vi "Simulate CNT90.vi"(8 "error in (no error)":errorcluster, 10 "frec in":dbl=0.75 format="%#_13g", 11 "VISA resource name":refnum<visa-resource-name>) -> (0 "error out":errorcluster, 2 "Simulated Measurement":dbl, 3 "VISA resource name out":refnum<visa-resource-name>)   [LabVIEW 2019, in "CNT90.lvlib"]
uses:
  CNT90.lvlib
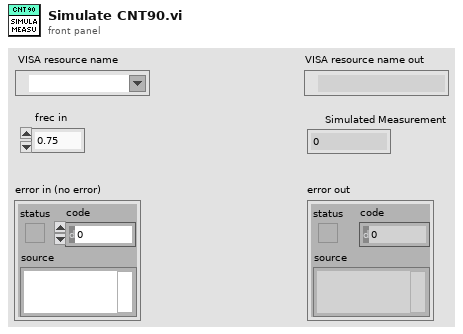
[diagram p1: front panel]
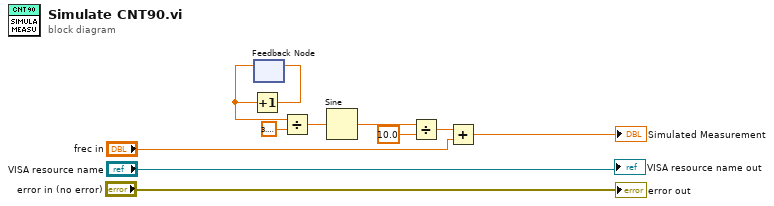
[diagram p0: block diagram]
diagram:
  n1 = feedback #1() -> (w7:dbl)  [unwired: 1 in]
  n2 = Increment(x=w7) -> (x+1=w11:dbl)
  n3 = feedback-in #1(w11) -> ()
  n4 = Divide(x=w7, y=3.141592653589793) -> (x/y=w10:dbl)
  n5 = Sine(x=w10) -> (sin(x)=w8:dbl)
  n6 = Divide(x=w8, y=10.0) -> (x/y=w6:dbl)
  n7 = Add(x=w6, y="frec in") -> (x+y=→"Simulated Measurement":dbl)
  "error out" <- "error in (no error)"
  "VISA resource name out" <- "VISA resource name"
